vi "Draw Border.vi"(8 "error in (no error)":errorcluster, 11 "Line in":refnum<class "Line.lvclass">) -> (0 "error out":errorcluster, 2 "Picture out":picture, 3 "Line out":refnum<class "Line.lvclass">)   [LabVIEW 2015, in "Line.lvclass"]
uses:
  Line.lvclass
  Line Border/Line Border.lvclass
  Graphic/Graphic.lvclass/Graphic.ctl
  Line Border/Line Border.lvclass/Line Border.ctl
  Scalable Border/Scalable Border.lvclass
  Graphic/Graphic.lvclass
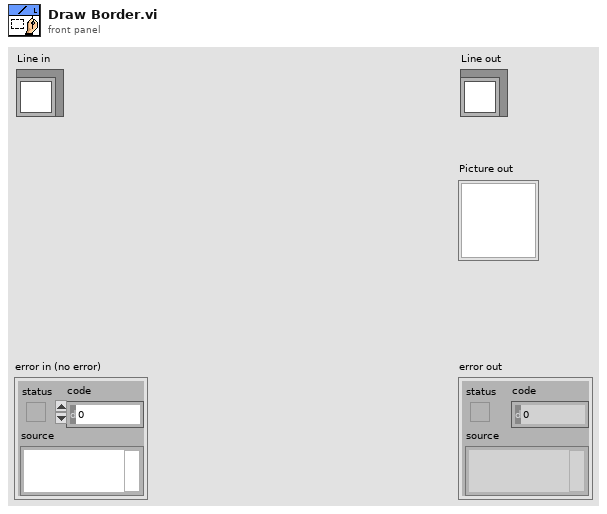
[diagram p1: front panel]
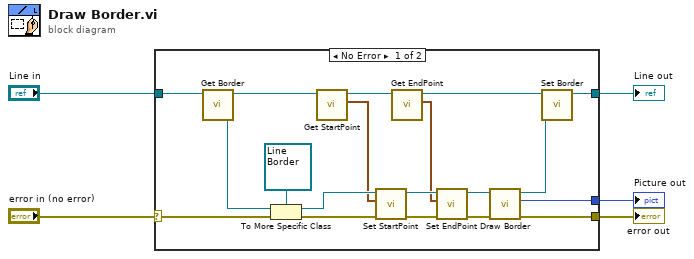
[diagram p0: block diagram]
diagram:
  n1 = case shown="No Error" "error in (no error)" {
    selector: "error in (no error)" -> [w15 w26]
    tunnel: "Line in" -> [w8 w25]
    tunnel: [w10 w25] -> w4
    tunnel: [w16 _] -> w3
    tunnel: [w14 w26] -> w1
    frame No Error {
      n2 = call "Get Border.vi"("Graphic in"=w8) -> ("Scalable Border.lvclass"=w23:refnum<class "Scalable Border.lvclass">, "Graphic out"=w7:refnum<class "Line.lvclass">)  [unwired: 8 in, 1 out]
      n3 = To More Specific Class(target class=refnum<class "Line Border.lvclass"> refnum ("Line Border.lvclass"), reference=w23, error in=w15) -> (specific class reference=w22:refnum<class "Line Border.lvclass">, error out=w20:errorcluster)
      n4 = call "Get StartPoint.vi"("Graphic in"=w7) -> ("StartPoint"=w13:cluster{"x":i16, "y":i16}, "Graphic out"=w12:refnum<class "Line.lvclass">)  [unwired: 8 in, 1 out]
      n5 = call "Set StartPoint.vi"("error in (no error)"=w20, "StartPoint"=w13, "Line Border in"=w22) -> ("error out"=w19:errorcluster, "Line Border out"=w21:refnum<class "Line Border.lvclass">)  [unwired: 7 in]
      n6 = call "Get EndPoint.vi"("Graphic in"=w12) -> ("EndPoint"=w11:cluster{"x":i16, "y":i16}, "Graphic out"=w6:refnum<class "Line.lvclass">)  [unwired: 8 in, 1 out]
      n7 = call "Set EndPoint.vi"("error in (no error)"=w19, "EndPoint"=w11, "Line Border in"=w21) -> ("error out"=w17:errorcluster, "Line Border out"=w18:refnum<class "Line Border.lvclass">)  [unwired: 7 in]
      n8 = call-dynamic "Draw Border.vi"("error in (no error)"=w17, "Line Border in"=w18) -> ("error out"=w14:errorcluster, "Border out"=w16:picture, "Line Border out"=w9:refnum<class "Line Border.lvclass">)  [unwired: 7 in]
      n9 = call "Set Border.vi"("Scalable Border.lvclass"=w9, "Graphic in"=w6) -> ("Graphic out"=w10:refnum<class "Line.lvclass">)  [unwired: 8 in, 1 out]
    }
    frame Error {
    }
  }
  "error out" <- w1
  "Line out" <- w4
  "Picture out" <- w3
